vi "VI Tree.vi"   [LabVIEW 2020, in "Marlin Instrument Driver.lvlib"]
doc: "This is the instrument driver for the <INSTRUMENT NAME>. The VI Tree displays all the user-callable VIs of the instrument driver in an organized table."
uses:
  <instrlib>/Marlin Instrument Driver/Marlin Instrument Driver.lvlib
panel:
  # "2021 Proper Printing.  ALL RIGHTS RESERVED."
  # "SEE DIAGRAM\nFOR VI TREE."
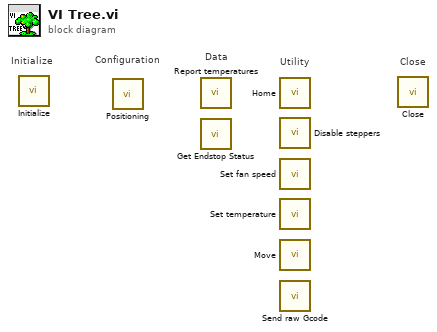
[diagram p0: block diagram]
diagram:
  # "Configuration"
  # "Utility"
  # "Data"
  # "Close"
  # "Initialize"
  n1 = call <instrlib>:"Initialize.vi"() -> ()  [unwired: 10 in, 2 out]
  n2 = call <instrlib>:"Positioning.vi"() -> ()  [unwired: 10 in, 2 out]
  n3 = call <instrlib>:"Report temperatures.vi"() -> ()  [unwired: 9 in, 3 out]
  n4 = call <instrlib>:"Get Endstop Status.vi"() -> ()  [unwired: 9 in, 3 out]
  n5 = call <instrlib>:"Home.vi"() -> ()  [unwired: 10 in, 2 out]
  n6 = call <instrlib>:"Disable steppers.vi"() -> ()  [unwired: 10 in, 2 out]
  n7 = call <instrlib>:"Set fan speed.vi"() -> ()  [unwired: 10 in, 2 out]
  n8 = call <instrlib>:"Set temperature.vi"() -> ()  [unwired: 10 in, 2 out]
  n9 = call <instrlib>:"Move.vi"() -> ()  [unwired: 10 in, 2 out]
  n10 = call <instrlib>:"Send raw Gcode.vi"() -> ()  [unwired: 8 in, 4 out]
  n11 = call <instrlib>:"Close.vi"() -> ()  [unwired: 11 in, 1 out]
